vi "HatchSideCollisionAvoidance.vi"(11 "Intended Hatch Setpoint":dbl) -> (3 "Modified Hatch Setpoint":dbl)   [LabVIEW 2018]
uses:
  Infrastructure/Constants.vi
  Robot Global Data.vi
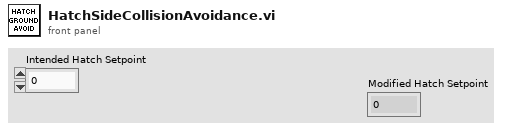
[diagram p1: front panel]
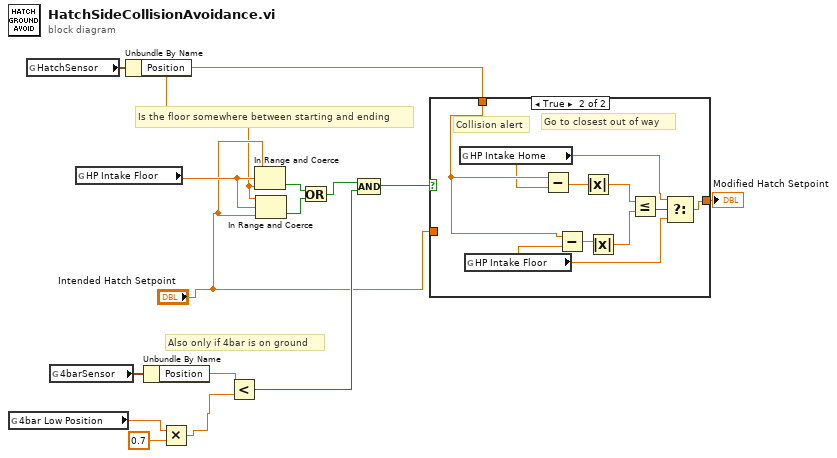
[diagram p0: block diagram]
diagram:
  # "Also only if 4bar is on ground"
  # "Is the floor somewhere between starting and ending"
  n1 = global read "Constants.vi" "4bar Low Position"() -> (w8:dbl)
  n2 = global read "Robot Global Data.vi" "HatchSensor"() -> (w15:cluster{"Position":dbl, "Velocity":dbl})
  n3 = global read "Robot Global Data.vi" "4barSensor"() -> (w13:cluster{"Position":dbl, "Velocity":dbl})
  n4 = global read "Constants.vi" "HP Intake Floor"() -> (w6:dbl)
  n5 = Unbundle By Name(w15) -> ("Position"=w1:dbl)
  n6 = Unbundle By Name(w13) -> ("Position"=w11:dbl)
  n7 = Multiply(x=w8, y=0.7) -> (x*y=w9:dbl)
  n8 = Less?(x=w11, y=w9) -> (x < y?=w10:bool)
  n9 = In Range and Coerce(upper limit="Intended Hatch Setpoint", x=w6, lower limit=w1) -> (In Range?=w4:bool)  [unwired: 1 out]
  n10 = In Range and Coerce(upper limit=w1, x=w6, lower limit="Intended Hatch Setpoint") -> (In Range?=w3:bool)  [unwired: 1 out]
  n11 = Or(x=w4, y=w3) -> (x .or. y?=w2:bool)
  n12 = Compound Arithmetic op=AND(w2, w10) -> (w12:bool)
  n13 = case shown="True" w12 {
    tunnel: [w16 w19] -> w14
    tunnel: "Intended Hatch Setpoint" -> [w16 _]
    tunnel: w1 -> [_ w25]
    frame False {
      # "Don't mess with it\nits good"
    }
    frame True {
      # "Go to closest out of way"
      # "Collision alert"
      n14 = global read "Constants.vi" "HP Intake Home"() -> (w17:dbl)
      n15 = global read "Constants.vi" "HP Intake Floor"() -> (w18:dbl)
      n16 = Subtract(x=w25, y=w17) -> (x-y=w24:dbl)
      n17 = Subtract(x=w25, y=w18) -> (x-y=w23:dbl)
      n18 = Absolute Value(x=w24) -> (abs(x)=w22:dbl)
      n19 = Absolute Value(x=w23) -> (abs(x)=w21:dbl)
      n20 = Less Or Equal?(x=w22, y=w21) -> (x <= y?=w20:bool)
      n21 = Select(t=w17, s=w20, f=w18) -> (s? t:f=w19:dbl)
    }
  }
  "Modified Hatch Setpoint" <- w14
